vi "Push Sync Files to WebDAV.vi"(0 "AKLH Sync Base":path, 5 "WebDAV IP":string="10.31.176.36", 7 "Sync Time (min)":i32, 9 "WebDAV Push":bool) -> ()   [LabVIEW 2018]
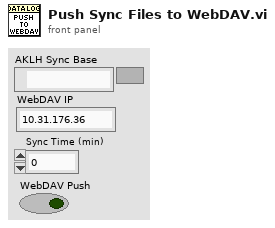
[diagram p1: front panel]
types:
  T1 = typedef "LVDateTimeRec.ctl" = cluster{"fractional second":dbl, "second":i32, "minute":i32, "hour":i32, "day of month":i32, "month":i32, "year":i32, "day of week":i32, "day of year":i32, "DST":i32}
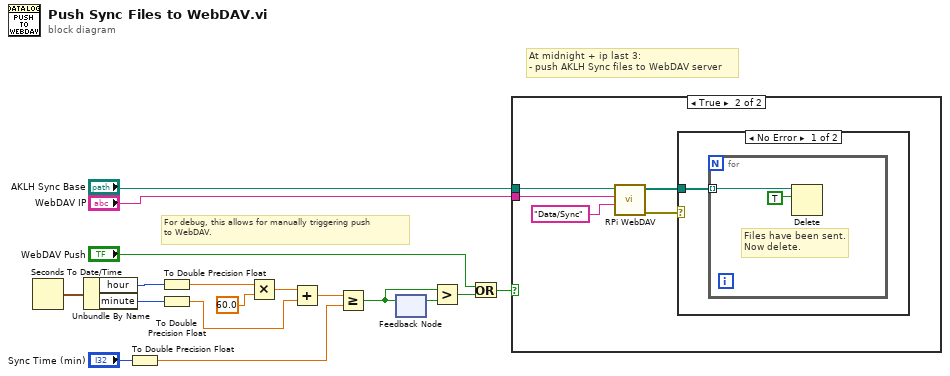
[diagram p0: block diagram]
diagram:
  # "For debug, this allows for manually triggering push\nto WebDAV."
  # "At midnight + ip last 3:\n- push AKLH Sync files to WebDAV server"
  n1 = Seconds To Date/Time() -> (date time rec=w15:T1)  [unwired: 2 in]
  n2 = Unbundle By Name(w15) -> ("hour"=w6:i32, "minute"=w12:i32)
  n3 = To Double Precision Float(number="Sync Time (min)") -> (double precision float=w7:dbl)
  n4 = To Double Precision Float(number=w6) -> (double precision float=w14:dbl)
  n5 = To Double Precision Float(number=w12) -> (double precision float=w10:dbl)
  n6 = Multiply(x=w14, y=60.0) -> (x*y=w11:dbl)
  n7 = Add(x=w11, y=w10) -> (x+y=w8:dbl)
  n8 = Greater Or Equal?(x=w8, y=w7) -> (x >= y?=w1:bool)
  n9 = feedback-in #1(w1) -> ()
  n10 = feedback #1() -> (w5:bool)  [unwired: 1 in]
  n11 = Greater?(x=w1, y=w5) -> (0:w4:bool)
  n12 = Or(x="WebDAV Push", y=w4) -> (x .or. y?=w2:bool)
  n13 = case shown="True" w2 {
    tunnel: "AKLH Sync Base" -> [_ w19]
    tunnel: "WebDAV IP" -> [_ w22]
    frame False {
    }
    frame True {
      n14 = call "RPi WebDAV.vi"("RPi Sub-Dir"="Data/Sync", "RPi IP"=w22, "RIO Folder"=w19) -> ("Error OUT"=w20:errorcluster, "Files Paths"=w18:path[])  [unwired: 7 in]
      n15 = case shown="No Error" w20 {
        tunnel: w18 -> [w23 _]
        frame No Error {
          n16 = for {
            tunnel: w23 -> [w25] mode=indexing
            # "Files have been sent.\nNow delete."
            n17 = Delete(path (use dialog)=w25, entire hierarchy (F)=TRUE ("confirm (F)")) -> ()  [unwired: 3 in, 3 out]
          }
        }
        frame Error {
          # "If error communicating with\nWebDAV, then leave the files\nalone and try tomorrow."
        }
      }
    }
  }
